vi "Hybrid Drive.vi"(6 "Async?":dbl, 8 "Max Accel":dbl, 9 "Max Velocity":dbl, 11 "Distance":dbl) -> (3 "Finished?":bool)   [LabVIEW 2015]
uses:
  Robot Global Data.vi
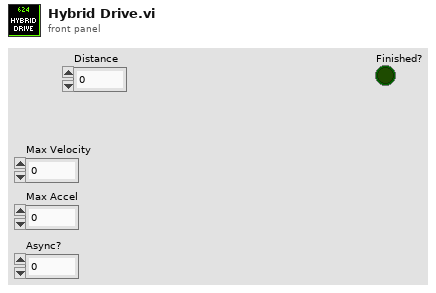
[diagram p1: front panel]
types:
  T1 = typedef "Drivetrain Status Cluster.ctl" = cluster{"Modes":T2, "Y (Throttle)":dbl, "X (Steer)":dbl, "Gyro In Range?":bool, "Distance Drive Finished?":bool, "Stop Eject Lockout":bool, "Dist Drive Status":T3, "Y Target":dbl, "Heading Target":dbl, "Vision Target Aligned?":bool, "Gear":dbl, "1st Gear Time":dbl, "2nd Gear Time":dbl, "1st Gear Shifts":dbl, "2nd Gear Shifts":dbl}
  T2 = typedef "Drivetrain Modes.ctl" = enum16{"Climb", "Manual", "Vision Targeting", "PID Distance Drive", "Hybrid"}
  T3 = typedef "Dist Drive Status.ctl" = cluster{"Y In Range":bool, "X In Range":bool, "Gyro In Range":bool, "Y Dist":dbl, "X Dist":dbl, "Gyro":dbl}
  T4 = typedef "Drivetrain Commands.ctl" = cluster{"Y Power":dbl, "Turn Power":dbl, "1st Gear?":bool, "Modes":T2, "Heading Target":dbl, "X Max Speed":dbl, "Y Max Speed":dbl, "X Min Speed":dbl, "Y Min Speed":dbl, "Y Target":dbl, "Max Accel":dbl, "Max Velocity":dbl}
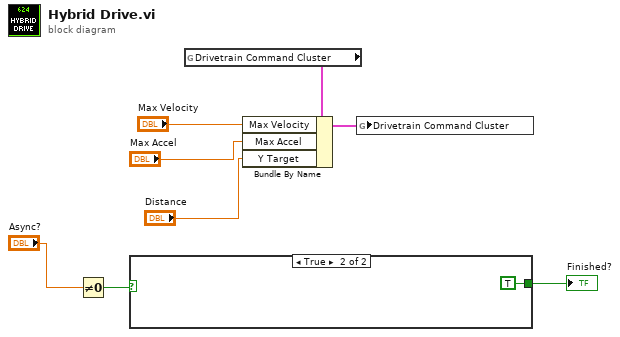
[diagram p0: block diagram]
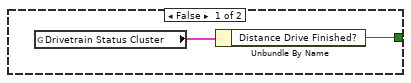
[diagram p2: hidden frame]
diagram:
  n1 = Not Equal To 0?(x="Async?") -> (x != 0?=w2:bool)
  n2 = case shown="True" w2 {
    tunnel: [w9 TRUE ("Distance Drive Finished?")] -> w3
    frame False {
      n3 = global read "Robot Global Data.vi" "Drivetrain Status Cluster"() -> (w10:T1)
      n4 = Unbundle By Name(w10) -> ("Distance Drive Finished?"=w9:bool)
    }
    frame True {
    }
  }
  "Finished?" <- w3
  n5 = global read "Robot Global Data.vi" "Drivetrain Command Cluster"() -> (w5:T4)
  n6 = Bundle By Name(cluster=w5, "Max Velocity"="Max Velocity", "Max Accel"="Max Accel", "Y Target"="Distance") -> (w6:T4)
  n7 = global write "Robot Global Data.vi" "Drivetrain Command Cluster"(w6) -> ()
